vi "PCO_ConvertSetSensorInfo.vi"(8 "error in (no error)":errorcluster {"code" format="%x"}, 10 "strSensorInfo":T1 {"iSensorInfoBits" items=["CONVERT_SENSOR_COLORIMAGE"=1, "CONVERT_SENSOR_UPPERALIGNED"=2]}, 11 "ph":u64) -> (0 "error out":errorcluster {"code" format="%x"}, 2 "ErrorMessage":i32 format="%x", 3 "ph out":u64)   [LabVIEW 2019, in "Convert.lvlib"]
doc: "int PCOCONVERT_API PCO_ConvertSetSensorInfo(HANDLE ph, PCO_SensorInfo* pstrSensorInfo);"
uses:
  Convert.lvlib
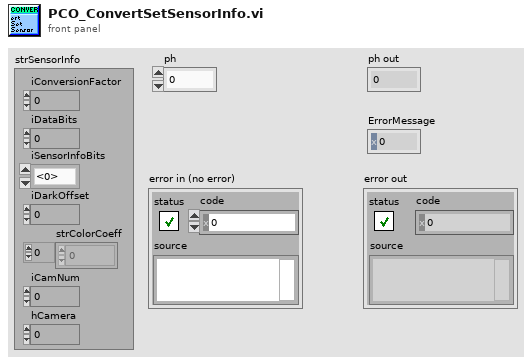
[diagram p1: front panel]
types:
  T1 = cluster{"iConversionFactor":i32, "iDataBits":i32, "iSensorInfoBits":i32, "iDarkOffset":i32, "strColorCoeff":dbl[], "iCamNum":i32, "hCamera":u64}
  T2 = cluster{"wSize":u16, "wDummy":u16, "iConversionFactor":i32, "iDataBits":i32, "iSensorInfoBits":i32, "iDarkOffset":i32, "dwzzDummy0":u32, "strColorCoeff":cluster{dbl, dbl, dbl, dbl, dbl, dbl, dbl, dbl, dbl}, "iCamNum":i32, "hCamera":u64, "dwzzDummy1":cluster{u32, u32, u32, u32, u32, u32, u32, u32, u32, u32, u32, u32, u32, u32, u32, u32, u32, u32, u32, u32, u32, u32, u32, u32, u32, u32, u32, u32, u32, u32, u32, u32, u32, u32, u32, u32, u32, u32, u32}}
  T3 = cluster{"wSize":u16, "wDummy":u16, "iConversionFactor":i32, "iDataBits":i32, "iSensorInfoBits":i32, "iDarkOffset":i32, "dwzzDummy0":u32, "strColorCoeff":cluster{dbl, dbl, dbl, dbl, dbl, dbl, dbl, dbl, dbl}, "iCamNum":i32, "hCamera":u32, "dwzzDummy1":cluster{u32, u32, u32, u32, u32, u32, u32, u32, u32, u32, u32, u32, u32, u32, u32, u32, u32, u32, u32, u32, u32, u32, u32, u32, u32, u32, u32, u32, u32, u32, u32, u32, u32, u32, u32, u32, u32, u32}}
  T4 = cluster{u32, u32, u32, u32, u32, u32, u32, u32, u32, u32, u32, u32, u32, u32, u32, u32, u32, u32, u32, u32, u32, u32, u32, u32, u32, u32, u32, u32, u32, u32, u32, u32, u32, u32, u32, u32, u32, u32, u32}
  T5 = cluster{"strColorCoeff[0]":dbl, "strColorCoeff[1]":dbl, "strColorCoeff[2]":dbl, "strColorCoeff[3]":dbl, "strColorCoeff[4]":dbl, "strColorCoeff[5]":dbl, "strColorCoeff[6]":dbl, "strColorCoeff[7]":dbl, "strColorCoeff[8]":dbl}
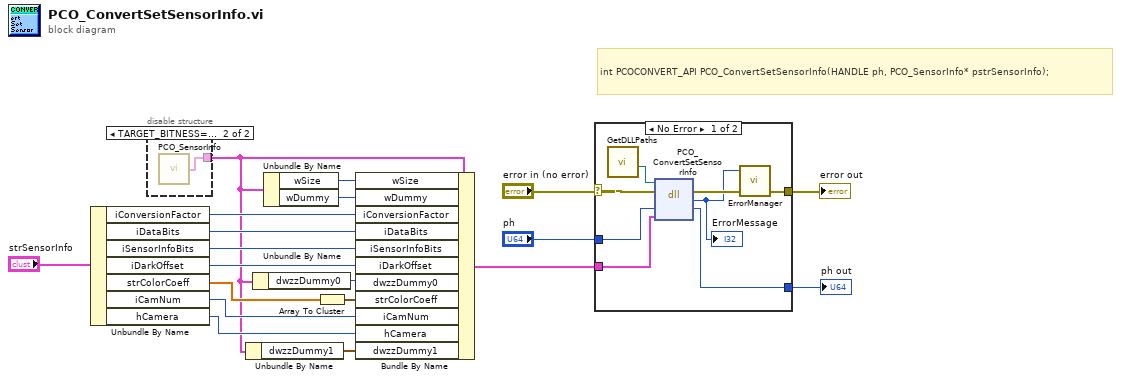
[diagram p0: block diagram]
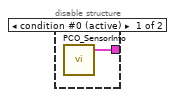
[diagram p2: hidden frame]
diagram:
  # "int PCOCONVERT_API PCO_ConvertSetSensorInfo(HANDLE ph, PCO_SensorInfo* pstrSensorInfo);"
  n1 = Unbundle By Name("strSensorInfo") -> ("iConversionFactor"=w14:i32, "iDataBits"=w13:i32, "iSensorInfoBits"=w12:i32, "iDarkOffset"=w11:i32, "strColorCoeff"=w10:dbl[], "iCamNum"=w8:i32, "hCamera"=w7:u64)
  n2 = disable-structure "Diagram Disable Structure" shown="TARGET_BITNESS==32" {
    disable-tunnel: [w20 w21] -> w2
    frame condition #0 (active) {
      n3 = call "PCO_SensorInfo.vi"() -> ("PCO_SensorInfo_Raw_x64"=w20:T2)  [unwired: 4 in, 4 out]
    }
    frame condition #1 {
      n4 = call "PCO_SensorInfo.vi"() -> ("PCO_SensorInfo_Raw_win32"=w21:T3)  [unwired: 4 in, 4 out]
    }
  }
  n5 = Unbundle By Name(w2) -> ("dwzzDummy1"=w6:T4)
  n6 = Unbundle By Name(w2) -> ("dwzzDummy0"=w1:u32)
  n7 = Unbundle By Name(w2) -> ("wSize"=w5:u16, "wDummy"=w4:u16)
  n8 = Array To Cluster(array=w10) -> (cluster=w9:T5)
  n9 = Bundle By Name(cluster=w2, "wSize"=w5, "wDummy"=w4, "iConversionFactor"=w14, "iDataBits"=w13, "iSensorInfoBits"=w12, "iDarkOffset"=w11, "dwzzDummy0"=w1, "strColorCoeff"=w9, "iCamNum"=w8, "hCamera"=w7, "dwzzDummy1"=w6) -> (w3:T2)
  n10 = case shown="No Error" "error in (no error)" {
    selector: "error in (no error)" -> [w27 w31]
    tunnel: "ph" -> [w29 w30]
    tunnel: [w28 w30] -> w18
    tunnel: [w25 w31] -> w17
    tunnel: w3 -> [w23 _]
    frame No Error {
      n11 = call "GetDLLPaths.vi"() -> ("PCO_Conv_Path"=w22:path)  [unwired: 9 in, 2 out]
      n12 = dll-call lib="?" fn="PCO_ConvertSetSensorInfo"(path in=w22, error in=w27, "ph"=w29, "pstrSensorInfo"=w23) -> (error out=w26:errorcluster, "return type"=w24:i32, "ph"=w28:u64)  [unwired: 2 in, 1 out]
      "ErrorMessage" <- w24
      n13 = call "ErrorManager.vi"("error in (no error)"=w26, "error code"=w24) -> ("error out"=w25:errorcluster)  [unwired: 3 in]
    }
    frame Error {
    }
  }
  "ph out" <- w18
  "error out" <- w17
